vi "MessageReceiver.vi"(0 "STOMP In":refnum<class "STOMP.lvclass">, 5 "error in (no error)":errorcluster) -> (14 "STOMP out":refnum<class "STOMP.lvclass">, 19 "error out":errorcluster)   [LabVIEW 2017, in "STOMP.lvclass"]
uses:
  STOMP.lvclass
panel:
  out "string":string
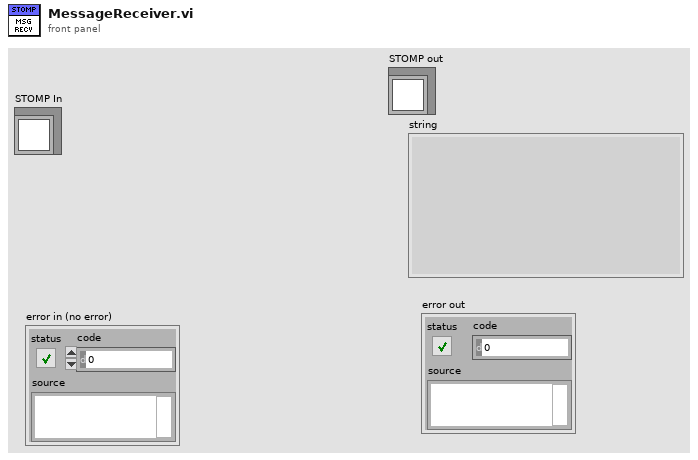
[diagram p1: front panel]
types:
  T1 = enum16{"Standard", "Buffered", "CRLF", "Immediate"}
  T2 = typedef "STOMP.lvclass/ObjectAttributes.ctl" = cluster{"address":string, "port":u16, "ConnectionRef":refnum<k5>, "messageQueue":refnum<queue>, "receiptQueue":refnum<queue>, "errorQueue":refnum<queue>, "sendQueue":refnum<queue>, "currentReceiptNumber":u64, "currentSubscriptionId":u64, "closeConnection":bool, "activeSubscriptions":T3[]}
  T3 = typedef "STOMP.lvclass/Type_ActiveSubscription.ctl" = cluster{"id":u64, "receipt":bool, "Destination":string, "ack":T4, "headers":T5[]}
  T4 = typedef "STOMP.lvclass/Type_AckHeader.ctl" = enum16{"auto", "client", "client-individual"}
  T5 = typedef "STOMP.lvclass/Type_FrameHeader.ctl" = cluster{"Header":string, "Value":string}
  T6 = typedef "STOMP.lvclass/Type_ServerFrame.ctl" = cluster{"Type":T7, "Headers":cluster{"Header":string, "Value":string}[], "Body":string}
  T7 = typedef "STOMP.lvclass/Type_ServerFrameType.ctl" = enum16{"Undefined", "MESSAGE", "CONNECTED", "RECEIPT", "ERROR"}
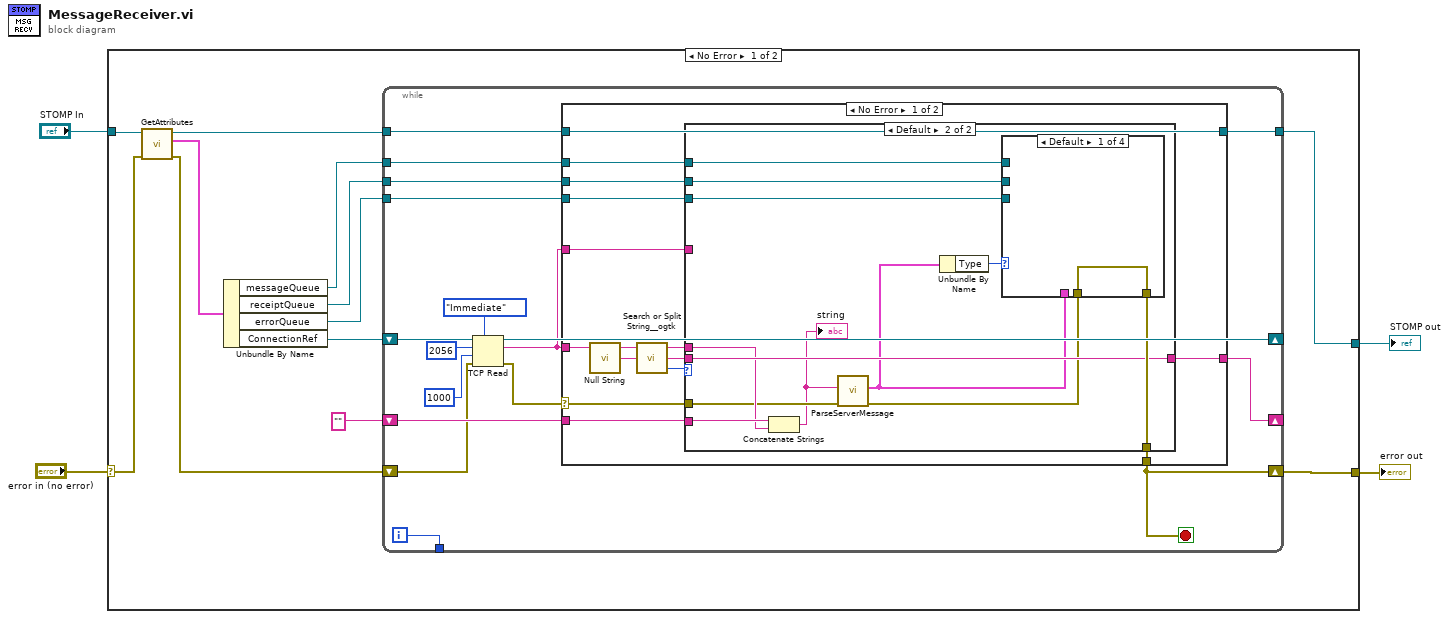
[diagram p0: block diagram]
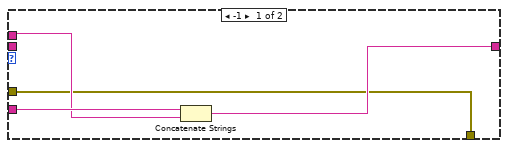
[diagram p2: hidden frame]
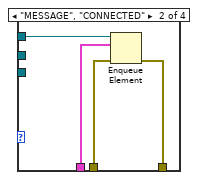
[diagram p3: hidden frame]
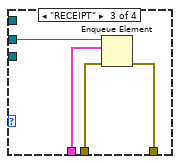
[diagram p4: hidden frame]
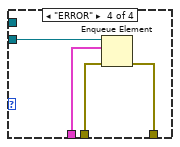
[diagram p5: hidden frame]
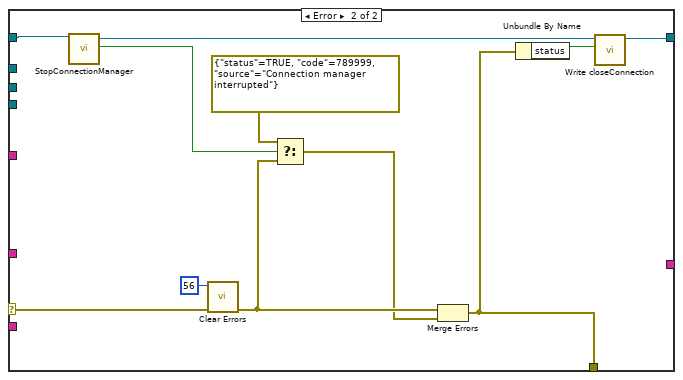
[diagram p6: hidden frame]
diagram:
  n1 = case shown="No Error" "error in (no error)" {
    selector: "error in (no error)" -> [w7 w89]
    tunnel: [w11 w89] -> w4
    tunnel: "STOMP In" -> [w9 w88]
    tunnel: [w10 w88] -> w2
    frame No Error {
      n2 = call-dynamic "GetAttributes.vi"("error in (no error)"=w7, "STOMP in"=w9) -> ("error out"=w6:errorcluster, "attributes"=w5:T2, "STOMP out"=w8:refnum<class "STOMP.lvclass">)  [unwired: 7 in]
      n3 = Unbundle By Name(w5) -> ("messageQueue"=w14:refnum<queue>, "receiptQueue"=w13:refnum<queue>, "errorQueue"=w12:refnum<queue>, "ConnectionRef"=w15:refnum<k5>)
      n4 = while {
        shift-right: [w30] -> _
        shift-left: w15 -> [w31]
        shift-right: [w25] -> _
        shift-left: "" -> [w29]
        tunnel: w14 -> [w28]
        tunnel: w13 -> [w24]
        tunnel: w12 -> [w23]
        tunnel: [w22] -> _
        shift-right: [w21] -> w11
        shift-left: w6 -> [w27]
        tunnel: w8 -> [w19]
        tunnel: [w18] -> w10
        i -> [w22]
        stop <- w21 stop-if-true
        n5 = TCP Read(connection ID=w31, bytes to read=2056, error in (no error)=w27, 7:T1."Immediate" ("mode (standard)"), 9:1000 ("timeout ms (25000)")) -> (connection ID out=w30:refnum<k5>, data out=w17:string, error out=w20:errorcluster)
        n6 = case shown="No Error" w20 {
          selector: w20 -> [w37 w86]
          tunnel: w17 -> [w35 _]
          tunnel: w29 -> [w47 _]
          tunnel: w28 -> [w46 _]
          tunnel: [w41 _] -> w25
          tunnel: w24 -> [w40 _]
          tunnel: w23 -> [w39 _]
          tunnel: [w38 w77] -> w21
          tunnel: w19 -> [w36 w85]
          tunnel: [w36 w79] -> w18
          tunnel: w17 -> [w34 _]
          frame No Error {
            n7 = call "Null String.vi"() -> ("NULL"=w45:string)  [unwired: 19 in]
            n8 = call <userlib>:"Search or Split String__ogtk.vi"("search string/char (-)"=w45, "string"=w35) -> ("offset after match"=w43:i32, "substring after match"=w42:string, "substring before match"=w44:string)  [unwired: 1 in]
            n9 = case shown="Default" w43 {
              tunnel: w47 -> [w51 w63]
              tunnel: w46 -> [_ w62]
              tunnel: w37 -> [w48 w58]
              tunnel: [w48 w61] -> w38
              tunnel: w44 -> [w50 w59]
              tunnel: w42 -> [_ w60]
              tunnel: [w49 w60] -> w41
              tunnel: w40 -> [_ w55]
              tunnel: w39 -> [_ w54]
              tunnel: w34 -> [_ _]
              frame -1 {
                n10 = Concatenate Strings(w51, w50) -> (w49:string)
              }
              frame Default {
                n11 = Concatenate Strings(w63, w59) -> (w52:string)
                "string" <- w52
                n12 = call "ParseServerMessage.vi"("error in (no error)"=w58, "msg"=w52) -> ("error out"=w57:errorcluster, "ServerFrame"=w53:T6)  [unwired: 8 in]
                n13 = Unbundle By Name(w53) -> ("Type"=w56:T7)
                n14 = case shown="Default" w56 {
                  tunnel: w62 -> [_ w68 _ _]
                  tunnel: [w64 w67 w72 w76] -> w61
                  tunnel: w57 -> [w64 w66 w71 w75]
                  tunnel: w55 -> [_ _ w70 _]
                  tunnel: w54 -> [_ _ _ w74]
                  tunnel: w53 -> [_ w65 w69 w73]
                  frame Default {
                  }
                  frame "MESSAGE", "CONNECTED" {
                    n15 = Enqueue Element(queue=w68, element=w65, error in (no error)=w66) -> (error out=w67:errorcluster)  [unwired: 1 in, 2 out]
                  }
                  frame "RECEIPT" {
                    n16 = Enqueue Element(queue=w70, element=w69, error in (no error)=w71) -> (error out=w72:errorcluster)  [unwired: 1 in, 2 out]
                  }
                  frame "ERROR" {
                    n17 = Enqueue Element(queue=w74, element=w73, error in (no error)=w75) -> (error out=w76:errorcluster)  [unwired: 1 in, 2 out]
                  }
                }
              }
            }
          }
          frame Error {
            n18 = call-dynamic "StopConnectionManager.vi"("STOMP in"=w85) -> ("STOMP out"=w80:refnum<class "STOMP.lvclass">, "stop?"=w84:bool)  [unwired: 16 in, 1 out]
            n19 = call <vilib>:"Clear Errors.vi"("error in (no error)"=w86, "specific error code to clear (0: all)"=56) -> ("error out"=w82:errorcluster)  [unwired: 4 in, 1 out]
            n20 = Select(t=errorcluster {"status"=TRUE, "code"=789999, "source"="Connection manager interrupted"} ("error constant"), s=w84, f=w82) -> (s? t:f=w81:errorcluster)
            n21 = Merge Errors(w82, w81) -> (w77:errorcluster)
            n22 = Unbundle By Name(w77) -> ("status"=w78:bool)
            n23 = call-dynamic "Write closeConnection.vi"("closeConnection"=w78, "STOMP in"=w80) -> ("STOMP out"=w79:refnum<class "STOMP.lvclass">)  [unwired: 8 in, 1 out]
          }
        }
      }
    }
    frame Error {
    }
  }
  "error out" <- w4
  "STOMP out" <- w2
